vi "autonSample.vi"(0 "Auton Array":dbl[][](array[numeric]), 5 "LeftEncoder":dbl, 7 "RightEncoder":dbl, 11 "MeasuredHeading":dbl) -> (4 "Left Drive":dbl, 6 "Right Drive":dbl, 8 "Ramp ACT motor":dbl, 10 "Harvester":dbl, 13 "Shooter motor output":dbl, 14 "Turret Rotation":dbl, 15 "Convyeor":dbl)   [LabVIEW 2011]
uses:
  Robot Global Data.vi
panel:
  out "Primitive ID":i16
  out "Tzero":i64
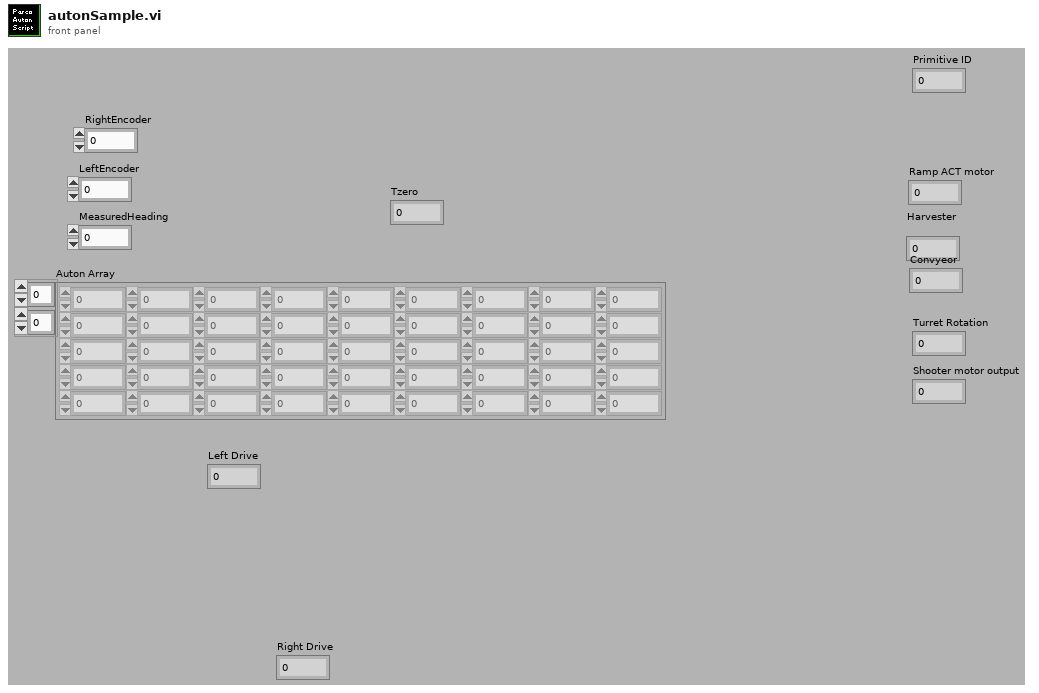
[diagram p1: front panel]
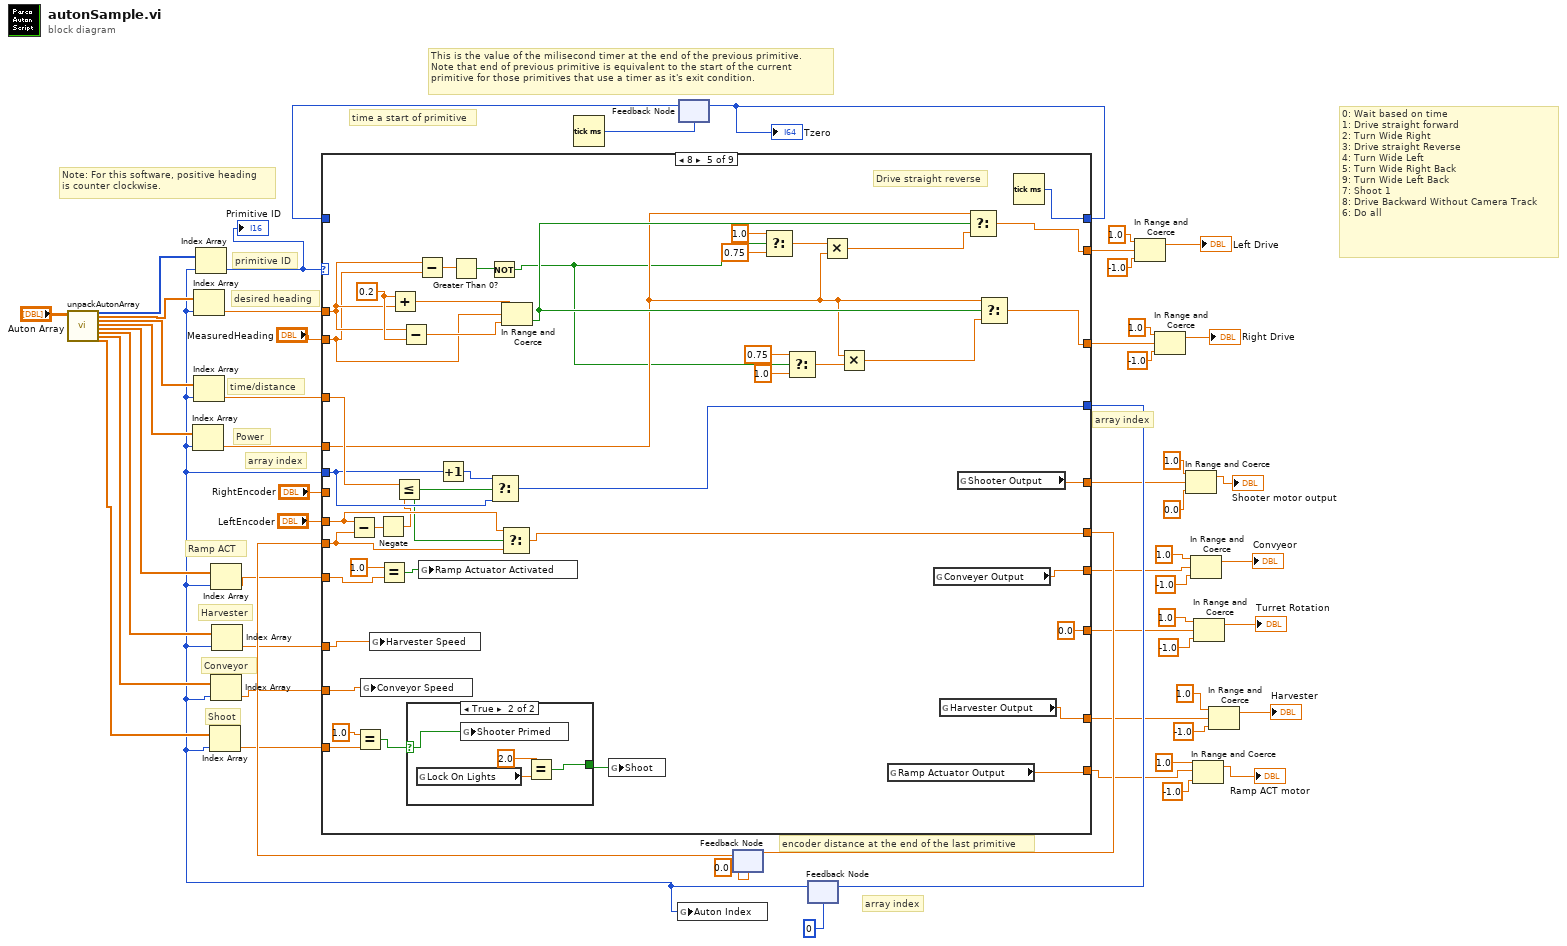
[diagram p0: block diagram]
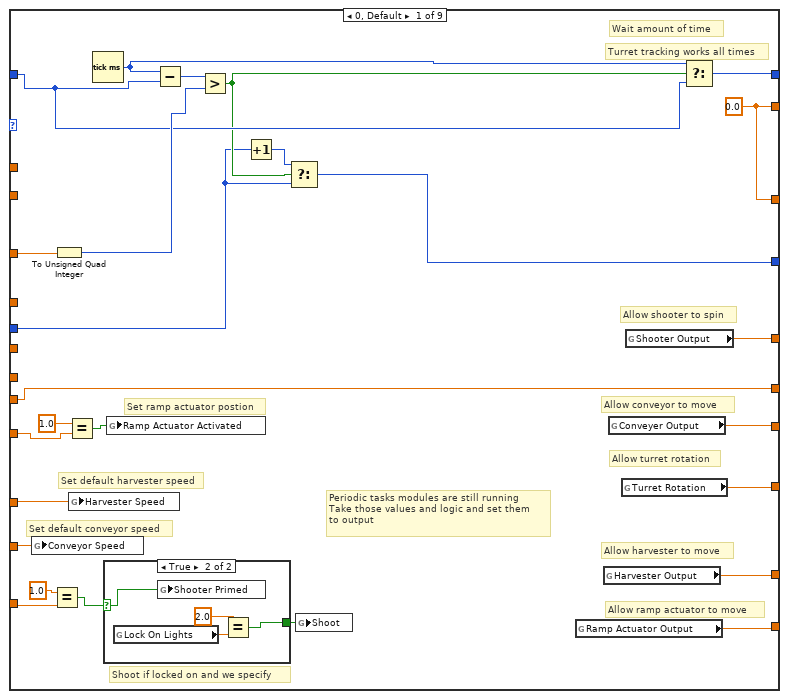
[diagram p2: hidden frame]
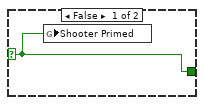
[diagram p3: hidden frame]
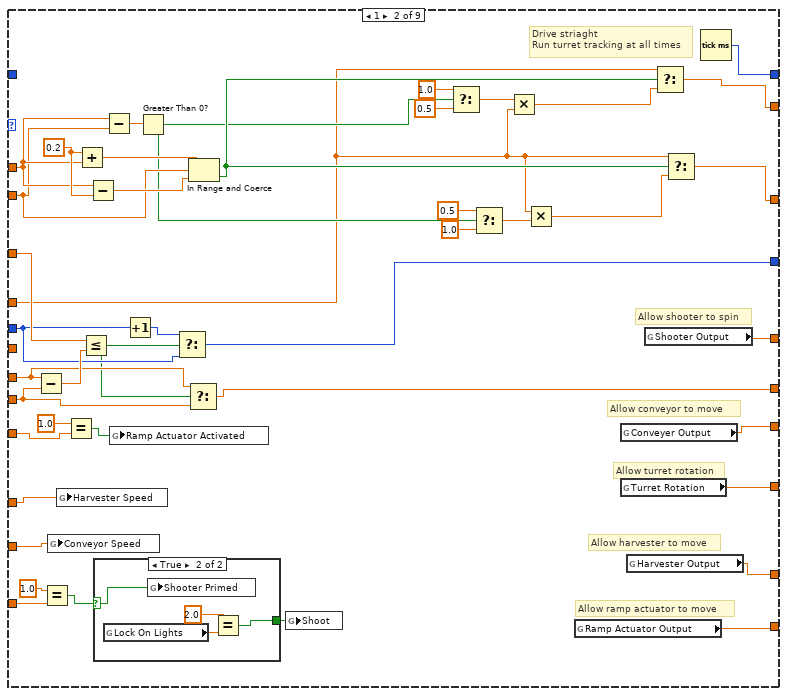
[diagram p4: hidden frame]
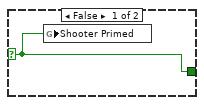
[diagram p5: hidden frame]
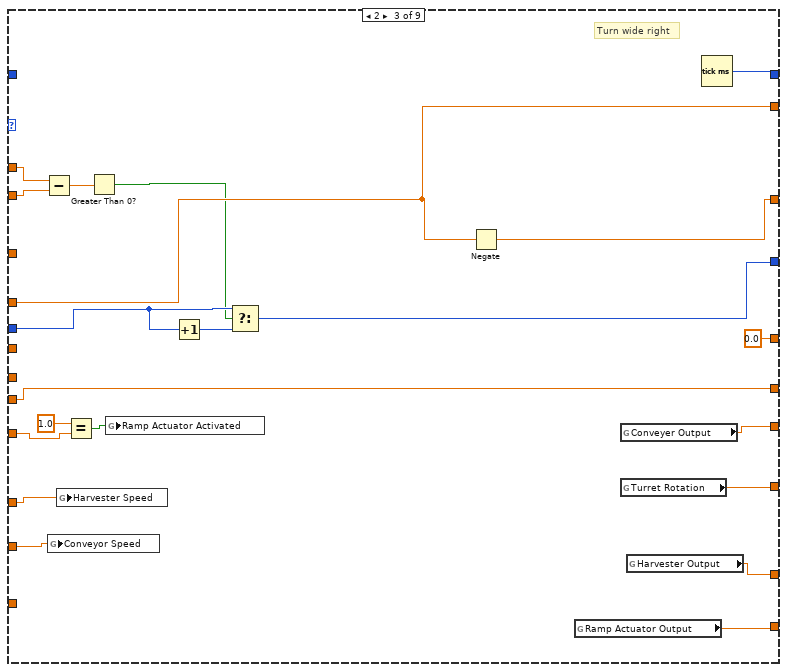
[diagram p6: hidden frame]
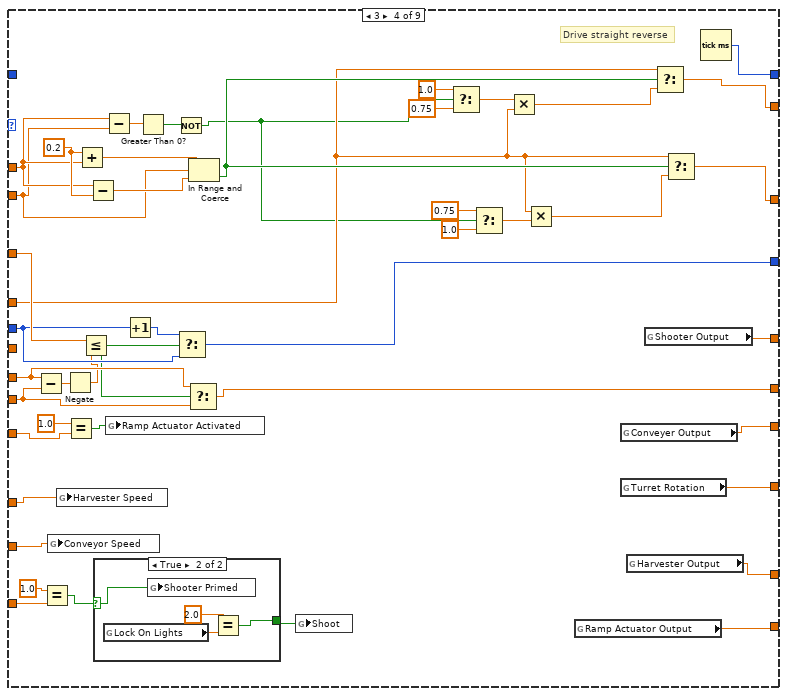
[diagram p7: hidden frame]
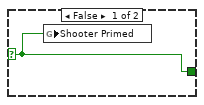
[diagram p8: hidden frame]
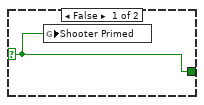
[diagram p9: hidden frame]
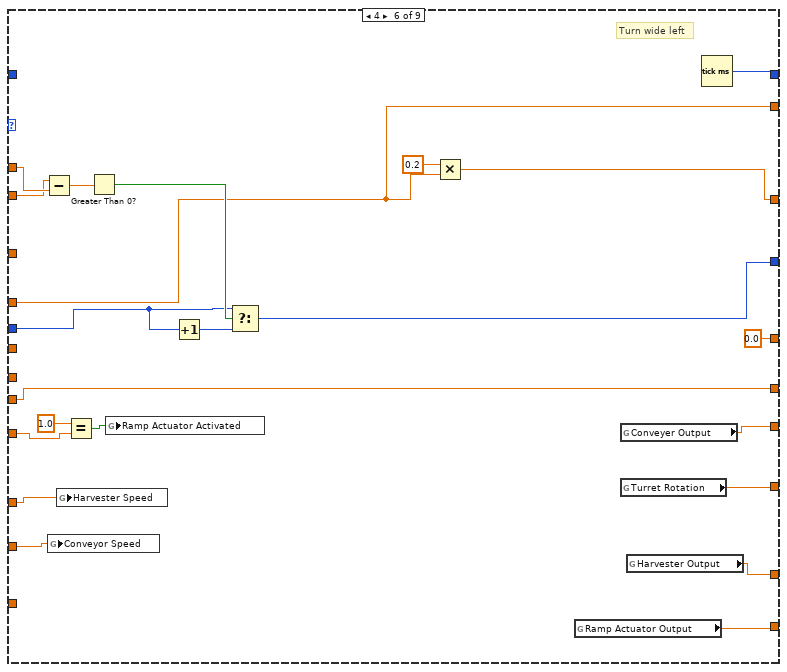
[diagram p10: hidden frame]
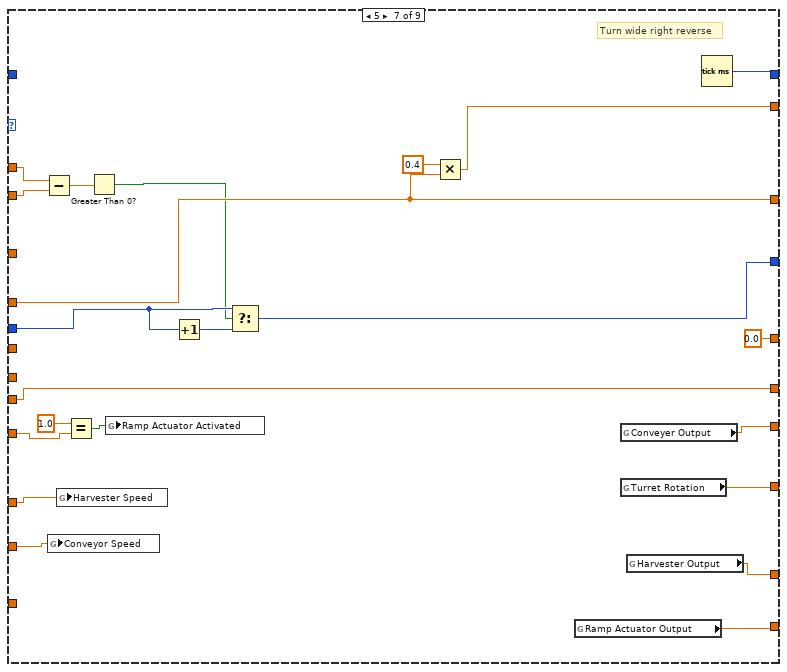
[diagram p11: hidden frame]
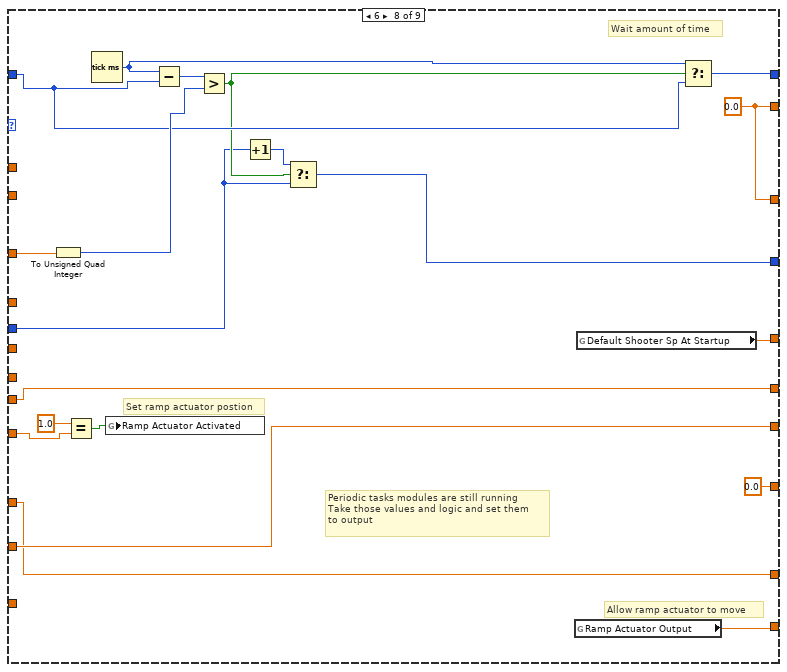
[diagram p12: hidden frame]
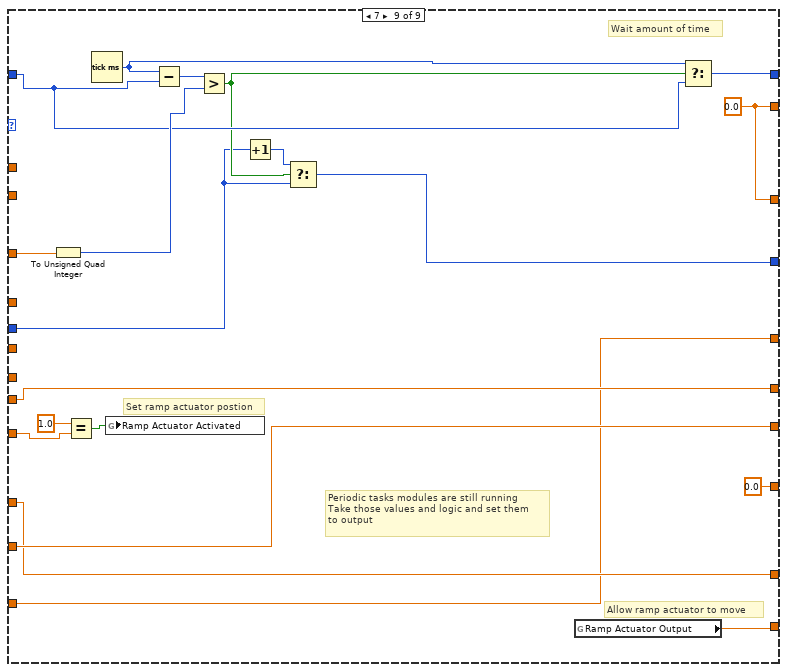
[diagram p13: hidden frame]
diagram:
  # "0: Wait based on time\n1: Drive straight forward\n2: Turn Wide Right\n3: Drive straight Reverse\n4: Turn Wide Left\n5: Turn Wide Right Back\n9: Turn Wide Left Back\n7: Shoot 1\n8: Drive Backward Without Camera Track\n6: Do all"
  # "Shoot"
  # "Conveyor"
  # "Harvester"
  # "Ramp ACT"
  # "encoder distance at the end of the last primitive"
  # "Note: For this software, positive heading\nis counter clockwise."
  # "time a start of primitive"
  # "array index"
  # "array index"
  # "This is the value of the milisecond timer at the end of the previous primitive.\nNote that end of previous primitive is equivalent to the start of the current\nprimitive for those primitives that use a timer as it's exit condition."
  # "Power"
  # "array index"
  # "desired heading"
  # "primitive ID"
  # "time/distance"
  n1 = call "unpackAutonArray.vi"("all rows"="Auton Array") -> ("Primitive"=w56:i16[], "Desired Heading"=w16:dbl[], "Time/Distance"=w15:dbl[], "Power"=w14:dbl[], "Ramp Actuator"=w13:dbl[], "Harvester"=w12:dbl[], "Conveyor"=w11:dbl[], "Shoot"=w10:dbl[])  [unwired: 1 in, 18 out]
  n2 = Tick Count (ms)() -> (millisecond timer value=w51:u32)
  n3 = feedback #1(w51) -> (w55:u32)
  n4 = feedback #2(0.0 ("EncoderDistance")) -> (w39:dbl)
  n5 = feedback #3(0) -> (w8:i32)
  n6 = Index Array(array=w14, index=w8) -> (element=w53:dbl)
  n7 = Index Array(array=w16, index=w8) -> (element=w40:dbl)
  n8 = Index Array(array=w15, index=w8) -> (element=w54:dbl)
  n9 = Index Array(array=w56, index=w8) -> (element=w22:i16)
  "Primitive ID" <- w22
  n10 = Index Array(array=w10, index=w8) -> (element=w9:dbl)
  n11 = Index Array(array=w13, index=w8) -> (element=w21:dbl)
  n12 = Index Array(array=w11, index=w8) -> (element=w6:dbl)
  n13 = Index Array(array=w12, index=w8) -> (element=w7:dbl)
  n14 = case shown="8" w22 {
    tunnel: [w75 w114 w140 w186 w237 w263 w281 w313 w333] -> w35
    tunnel: w8 -> [w76 w116 w142 w188 w239 w265 w283 w314 w334]
    tunnel: [w83 w92 w146 w165 w216 w269 w290 w321 w341] -> w41
    tunnel: w55 -> [w80 _ _ _ _ _ _ w318 w338]
    tunnel: w54 -> [w69 w117 _ w189 w240 _ _ w308 w328]
    tunnel: w40 -> [_ w105 w145 w177 w228 w260 w289 _ _]
    tunnel: [w74 w91 w139 w164 w215 w262 w285 w312 w332] -> w49
    tunnel: [w74 w90 w138 w163 w214 w261 w287 w312 w332] -> w42
    tunnel: w53 -> [_ w94 w139 w167 w218 w262 w287 _ _]
    tunnel: "LeftEncoder" -> [_ w111 _ w183 w234 _ _ _ _]
    tunnel: "MeasuredHeading" -> [_ w104 w144 w176 w227 w259 w288 _ _]
    tunnel: [w68 w113 w148 w185 w236 w271 w292 w307 w327] -> w36
    tunnel: w39 -> [w68 w112 w148 w184 w235 w271 w292 w307 w327]
    tunnel: [w58 w119 0.0 ("Shooter Output") w190 w241 0.0 ("Shooter Output") 0.0 ("Shooter Output") w302 w322] -> w31
    tunnel: [w70 w129 w154 w199 0.0 ("Turret Rotation") w276 w298 0.0 ("Turret Rotation") 0.0 ("Turret Rotation")] -> w27
    tunnel: [w66 w123 w150 w194 w245 w273 w294 w304 w324] -> w23
    tunnel: w21 -> [w63 w126 w153 w162 w213 w258 w297 w306 w326]
    tunnel: [w71 w130 w155 w200 w250 w277 w299 w309 w329] -> w20
    tunnel: w9 -> [w59 w127 _ w197 w248 _ _ _ w322]
    tunnel: w7 -> [w64 w125 w152 w196 w247 w275 w296 w304 w324]
    tunnel: w6 -> [w65 w124 w151 w195 w246 w274 w295 w305 w325]
    tunnel: [w67 w122 w149 w193 w244 w272 w293 w305 w325] -> w2
    tunnel: "RightEncoder" -> [_ _ _ _ _ _ _ _ _]
    frame 0, Default {
      w74 = 0.0 ("Numeric")
      # "Periodic tasks modules are still running\nTake those values and logic and set them \nto output"
      # "Set ramp actuator postion"
      # "Set default harvester speed"
      # "Set default conveyor speed"
      # "Shoot if locked on and we specify"
      # "Allow ramp actuator to move"
      # "Allow harvester to move"
      # "Turret tracking works all times"
      # "Allow turret rotation"
      # "Allow conveyor to move"
      # "Allow shooter to spin"
      # "Wait amount of time"
      n15 = global write "Robot Global Data.vi" "Conveyor Speed"(w65) -> ()
      n16 = Equal?(x=1.0, y=w59) -> (x = y?=w61:bool)
      n17 = To Unsigned Quad Integer(1:w69) -> (0:w81:u64)
      n18 = Equal?(x=1.0, y=w63) -> (x = y?=w72:bool)
      n19 = global write "Robot Global Data.vi" "Harvester Speed"(w64) -> ()
      n20 = Tick Count (ms)() -> (millisecond timer value=w79:u32)
      n21 = case shown="True" w61 {
        selector: w61 -> [w84 w88]
        tunnel: [w84 w85] -> w60
        frame False {
          n22 = global write "Robot Global Data.vi" "Shooter Primed"(w84) -> ()
        }
        frame True {
          n23 = global read "Robot Global Data.vi" "Lock On Lights"() -> (w86:dbl)
          n24 = global write "Robot Global Data.vi" "Shooter Primed"(w88) -> ()
          n25 = Equal?(x=2.0, y=w86) -> (x = y?=w85:bool)
        }
      }
      n26 = global write "Robot Global Data.vi" "Ramp Actuator Activated"(w72) -> ()
      n27 = Subtract(x=w79, y=w80) -> (x-y=w82:u32)
      n28 = Greater?(x=w82, y=w81) -> (0:w78:bool)
      n29 = Increment(x=w76) -> (x+1=w77:i32)
      n30 = Select(t=w77, s=w78, f=w76) -> (s? t:f=w75:i32)
      n31 = global write "Robot Global Data.vi" "Shoot"(w60) -> ()
      n32 = global read "Robot Global Data.vi" "Ramp Actuator Output"() -> (w71:dbl)
      n33 = global read "Robot Global Data.vi" "Harvester Output"() -> (w66:dbl)
      n34 = global read "Robot Global Data.vi" "Conveyer Output"() -> (w67:dbl)
      n35 = global read "Robot Global Data.vi" "Turret Rotation"() -> (w70:dbl)
      n36 = global read "Robot Global Data.vi" "Shooter Output"() -> (w58:dbl)
      n37 = Select(t=w79, s=w78, f=w80) -> (s? t:f=w83:u32)
    }
    frame 1 {
      w109 = 0.2 ("x")
      # "Allow ramp actuator to move"
      # "Allow harvester to move"
      # "Allow turret rotation"
      # "Allow conveyor to move"
      # "Allow shooter to spin"
      # "Drive striaght\nRun turret tracking at all times"
      n38 = Subtract(x=w111, y=w112) -> (x-y=w118:dbl)
      n39 = Equal?(x=1.0, y=w127) -> (x = y?=w121:bool)
      n40 = global write "Robot Global Data.vi" "Conveyor Speed"(w124) -> ()
      n41 = global write "Robot Global Data.vi" "Harvester Speed"(w125) -> ()
      n42 = Equal?(x=1.0, y=w126) -> (x = y?=w89:bool)
      n43 = Add(x=w109, y=w105) -> (x+y=w107:dbl)
      n44 = Less Or Equal?(x=w117, y=w118) -> (x <= y?=w110:bool)
      n45 = Subtract(x=w105, y=w109) -> (x-y=w108:dbl)
      n46 = case shown="True" w121 {
        selector: w121 -> [w132 w136]
        tunnel: [w132 w133] -> w120
        frame False {
          n47 = global write "Robot Global Data.vi" "Shooter Primed"(w132) -> ()
        }
        frame True {
          n48 = global read "Robot Global Data.vi" "Lock On Lights"() -> (w134:dbl)
          n49 = global write "Robot Global Data.vi" "Shooter Primed"(w136) -> ()
          n50 = Equal?(x=2.0, y=w134) -> (x = y?=w133:bool)
        }
      }
      n51 = Subtract(x=w105, y=w104) -> (x-y=w103:dbl)
      n52 = global write "Robot Global Data.vi" "Ramp Actuator Activated"(w89) -> ()
      n53 = Increment(x=w116) -> (x+1=w115:i32)
      n54 = Greater Than 0?(x=w103) -> (x > 0?=w102:bool)
      n55 = Select(t=w115, s=w110, f=w116) -> (s? t:f=w114:i32)
      n56 = Select(t=w111, s=w110, f=w112) -> (s? t:f=w113:dbl)
      n57 = In Range and Coerce(upper limit=w107, x=w104, lower limit=w108) -> (In Range?=w106:bool)  [unwired: 1 out]
      n58 = global write "Robot Global Data.vi" "Shoot"(w120) -> ()
      n59 = Select(t=1.0, s=w102, f=0.5) -> (s? t:f=w95:dbl)
      n60 = Select(t=0.5, s=w102, f=1.0) -> (s? t:f=w97:dbl)
      n61 = Multiply(x=w95, y=w94) -> (x*y=w93:dbl)
      n62 = Multiply(x=w94, y=w97) -> (x*y=w96:dbl)
      n63 = global read "Robot Global Data.vi" "Ramp Actuator Output"() -> (w130:dbl)
      n64 = global read "Robot Global Data.vi" "Conveyer Output"() -> (w122:dbl)
      n65 = global read "Robot Global Data.vi" "Turret Rotation"() -> (w129:dbl)
      n66 = global read "Robot Global Data.vi" "Harvester Output"() -> (w123:dbl)
      n67 = global read "Robot Global Data.vi" "Shooter Output"() -> (w119:dbl)
      n68 = Select(t=w94, s=w106, f=w93) -> (s? t:f=w91:dbl)
      n69 = Select(t=w94, s=w106, f=w96) -> (s? t:f=w90:dbl)
      n70 = Tick Count (ms)() -> (millisecond timer value=w92:u32)
    }
    frame 2 {
      # "Turn wide right"
      n71 = Subtract(x=w145, y=w144) -> (x-y=w143:dbl)
      n72 = global write "Robot Global Data.vi" "Conveyor Speed"(w151) -> ()
      n73 = global write "Robot Global Data.vi" "Harvester Speed"(w152) -> ()
      n74 = Equal?(x=1.0, y=w153) -> (x = y?=w156:bool)
      n75 = Greater Than 0?(x=w143) -> (x > 0?=w137:bool)
      n76 = global write "Robot Global Data.vi" "Ramp Actuator Activated"(w156) -> ()
      n77 = Increment(x=w142) -> (x+1=w141:i32)
      n78 = Select(t=w142, s=w137, f=w141) -> (s? t:f=w140:i32)
      n79 = Negate(x=w139) -> (-x=w138:dbl)
      n80 = global read "Robot Global Data.vi" "Ramp Actuator Output"() -> (w155:dbl)
      n81 = global read "Robot Global Data.vi" "Conveyer Output"() -> (w149:dbl)
      n82 = global read "Robot Global Data.vi" "Turret Rotation"() -> (w154:dbl)
      n83 = global read "Robot Global Data.vi" "Harvester Output"() -> (w150:dbl)
      n84 = Tick Count (ms)() -> (millisecond timer value=w146:u32)
    }
    frame 3 {
      w181 = 0.2 ("x")
      # "Drive straight reverse"
      n85 = Subtract(x=w183, y=w184) -> (x-y=w161:dbl)
      n86 = Equal?(x=1.0, y=w197) -> (x = y?=w192:bool)
      n87 = global write "Robot Global Data.vi" "Conveyor Speed"(w195) -> ()
      n88 = global write "Robot Global Data.vi" "Harvester Speed"(w196) -> ()
      n89 = Negate(x=w161) -> (-x=w160:dbl)
      n90 = Equal?(x=1.0, y=w162) -> (x = y?=w201:bool)
      n91 = Add(x=w181, y=w177) -> (x+y=w179:dbl)
      n92 = Less Or Equal?(x=w189, y=w160) -> (x <= y?=w182:bool)
      n93 = Subtract(x=w177, y=w181) -> (x-y=w180:dbl)
      n94 = case shown="True" w192 {
        selector: w192 -> [w203 w207]
        tunnel: [w203 w204] -> w191
        frame False {
          n95 = global write "Robot Global Data.vi" "Shooter Primed"(w203) -> ()
        }
        frame True {
          n96 = global read "Robot Global Data.vi" "Lock On Lights"() -> (w205:dbl)
          n97 = global write "Robot Global Data.vi" "Shooter Primed"(w207) -> ()
          n98 = Equal?(x=2.0, y=w205) -> (x = y?=w204:bool)
        }
      }
      n99 = Subtract(x=w177, y=w176) -> (x-y=w175:dbl)
      n100 = global write "Robot Global Data.vi" "Ramp Actuator Activated"(w201) -> ()
      n101 = Increment(x=w188) -> (x+1=w187:i32)
      n102 = Greater Than 0?(x=w175) -> (x > 0?=w159:bool)
      n103 = Not(x=w159) -> (.not. x?=w158:bool)
      n104 = Select(t=w187, s=w182, f=w188) -> (s? t:f=w186:i32)
      n105 = Select(t=w183, s=w182, f=w184) -> (s? t:f=w185:dbl)
      n106 = In Range and Coerce(upper limit=w179, x=w176, lower limit=w180) -> (In Range?=w178:bool)  [unwired: 1 out]
      n107 = global write "Robot Global Data.vi" "Shoot"(w191) -> ()
      n108 = Select(t=1.0, s=w158, f=0.75) -> (s? t:f=w168:dbl)
      n109 = Select(t=0.75, s=w158, f=1.0) -> (s? t:f=w170:dbl)
      n110 = Multiply(x=w168, y=w167) -> (x*y=w166:dbl)
      n111 = Multiply(x=w167, y=w170) -> (x*y=w169:dbl)
      n112 = global read "Robot Global Data.vi" "Ramp Actuator Output"() -> (w200:dbl)
      n113 = global read "Robot Global Data.vi" "Conveyer Output"() -> (w193:dbl)
      n114 = global read "Robot Global Data.vi" "Turret Rotation"() -> (w199:dbl)
      n115 = global read "Robot Global Data.vi" "Harvester Output"() -> (w194:dbl)
      n116 = global read "Robot Global Data.vi" "Shooter Output"() -> (w190:dbl)
      n117 = Select(t=w167, s=w178, f=w166) -> (s? t:f=w164:dbl)
      n118 = Select(t=w167, s=w178, f=w169) -> (s? t:f=w163:dbl)
      n119 = Tick Count (ms)() -> (millisecond timer value=w165:u32)
    }
    frame 8 {
      w232 = 0.2 ("x")
      # "Drive straight reverse"
      n120 = Subtract(x=w234, y=w235) -> (x-y=w212:dbl)
      n121 = Equal?(x=1.0, y=w248) -> (x = y?=w243:bool)
      n122 = global write "Robot Global Data.vi" "Conveyor Speed"(w246) -> ()
      n123 = global write "Robot Global Data.vi" "Harvester Speed"(w247) -> ()
      n124 = Negate(x=w212) -> (-x=w211:dbl)
      n125 = Equal?(x=1.0, y=w213) -> (x = y?=w251:bool)
      n126 = Add(x=w232, y=w228) -> (x+y=w230:dbl)
      n127 = Less Or Equal?(x=w240, y=w211) -> (x <= y?=w233:bool)
      n128 = Subtract(x=w228, y=w232) -> (x-y=w231:dbl)
      n129 = case shown="True" w243 {
        selector: w243 -> [w253 w257]
        tunnel: [w253 w254] -> w242
        frame False {
          n130 = global write "Robot Global Data.vi" "Shooter Primed"(w253) -> ()
        }
        frame True {
          n131 = global read "Robot Global Data.vi" "Lock On Lights"() -> (w255:dbl)
          n132 = global write "Robot Global Data.vi" "Shooter Primed"(w257) -> ()
          n133 = Equal?(x=2.0, y=w255) -> (x = y?=w254:bool)
        }
      }
      n134 = Subtract(x=w228, y=w227) -> (x-y=w226:dbl)
      n135 = global write "Robot Global Data.vi" "Ramp Actuator Activated"(w251) -> ()
      n136 = Increment(x=w239) -> (x+1=w238:i32)
      n137 = Greater Than 0?(x=w226) -> (x > 0?=w210:bool)
      n138 = Not(x=w210) -> (.not. x?=w209:bool)
      n139 = Select(t=w238, s=w233, f=w239) -> (s? t:f=w237:i32)
      n140 = Select(t=w234, s=w233, f=w235) -> (s? t:f=w236:dbl)
      n141 = In Range and Coerce(upper limit=w230, x=w227, lower limit=w231) -> (In Range?=w229:bool)  [unwired: 1 out]
      n142 = global write "Robot Global Data.vi" "Shoot"(w242) -> ()
      n143 = Select(t=1.0, s=w209, f=0.75) -> (s? t:f=w219:dbl)
      n144 = Select(t=0.75, s=w209, f=1.0) -> (s? t:f=w221:dbl)
      n145 = Multiply(x=w219, y=w218) -> (x*y=w217:dbl)
      n146 = Multiply(x=w218, y=w221) -> (x*y=w220:dbl)
      n147 = global read "Robot Global Data.vi" "Ramp Actuator Output"() -> (w250:dbl)
      n148 = global read "Robot Global Data.vi" "Conveyer Output"() -> (w244:dbl)
      n149 = global read "Robot Global Data.vi" "Harvester Output"() -> (w245:dbl)
      n150 = global read "Robot Global Data.vi" "Shooter Output"() -> (w241:dbl)
      n151 = Select(t=w218, s=w229, f=w217) -> (s? t:f=w215:dbl)
      n152 = Select(t=w218, s=w229, f=w220) -> (s? t:f=w214:dbl)
      n153 = Tick Count (ms)() -> (millisecond timer value=w216:u32)
    }
    frame 4 {
      # "Turn wide left"
      n154 = Subtract(x=w259, y=w260) -> (x-y=w267:dbl)
      n155 = global write "Robot Global Data.vi" "Conveyor Speed"(w274) -> ()
      n156 = global write "Robot Global Data.vi" "Harvester Speed"(w275) -> ()
      n157 = Equal?(x=1.0, y=w258) -> (x = y?=w278:bool)
      n158 = Greater Than 0?(x=w267) -> (x > 0?=w266:bool)
      n159 = global write "Robot Global Data.vi" "Ramp Actuator Activated"(w278) -> ()
      n160 = Increment(x=w265) -> (x+1=w264:i32)
      n161 = Select(t=w265, s=w266, f=w264) -> (s? t:f=w263:i32)
      n162 = Multiply(x=0.2, y=w262) -> (x*y=w261:dbl)
      n163 = global read "Robot Global Data.vi" "Ramp Actuator Output"() -> (w277:dbl)
      n164 = global read "Robot Global Data.vi" "Conveyer Output"() -> (w272:dbl)
      n165 = global read "Robot Global Data.vi" "Turret Rotation"() -> (w276:dbl)
      n166 = global read "Robot Global Data.vi" "Harvester Output"() -> (w273:dbl)
      n167 = Tick Count (ms)() -> (millisecond timer value=w269:u32)
    }
    frame 5 {
      # "Turn wide right reverse"
      n168 = Subtract(x=w289, y=w288) -> (x-y=w284:dbl)
      n169 = global write "Robot Global Data.vi" "Conveyor Speed"(w295) -> ()
      n170 = global write "Robot Global Data.vi" "Harvester Speed"(w296) -> ()
      n171 = Equal?(x=1.0, y=w297) -> (x = y?=w300:bool)
      n172 = Greater Than 0?(x=w284) -> (x > 0?=w280:bool)
      n173 = global write "Robot Global Data.vi" "Ramp Actuator Activated"(w300) -> ()
      n174 = Increment(x=w283) -> (x+1=w282:i32)
      n175 = Select(t=w283, s=w280, f=w282) -> (s? t:f=w281:i32)
      n176 = Multiply(x=0.4, y=w287) -> (x*y=w285:dbl)
      n177 = global read "Robot Global Data.vi" "Ramp Actuator Output"() -> (w299:dbl)
      n178 = global read "Robot Global Data.vi" "Conveyer Output"() -> (w293:dbl)
      n179 = global read "Robot Global Data.vi" "Turret Rotation"() -> (w298:dbl)
      n180 = global read "Robot Global Data.vi" "Harvester Output"() -> (w294:dbl)
      n181 = Tick Count (ms)() -> (millisecond timer value=w290:u32)
    }
    frame 6 {
      w312 = 0.0 ("Numeric")
      # "Periodic tasks modules are still running\nTake those values and logic and set them \nto output"
      # "Set ramp actuator postion"
      # "Allow ramp actuator to move"
      # "Wait amount of time"
      n182 = To Unsigned Quad Integer(1:w308) -> (0:w319:u64)
      n183 = Equal?(x=1.0, y=w306) -> (x = y?=w310:bool)
      n184 = Tick Count (ms)() -> (millisecond timer value=w317:u32)
      n185 = global write "Robot Global Data.vi" "Ramp Actuator Activated"(w310) -> ()
      n186 = Subtract(x=w317, y=w318) -> (x-y=w320:u32)
      n187 = Greater?(x=w320, y=w319) -> (0:w316:bool)
      n188 = Increment(x=w314) -> (x+1=w315:i32)
      n189 = Select(t=w315, s=w316, f=w314) -> (s? t:f=w313:i32)
      n190 = global read "Robot Global Data.vi" "Ramp Actuator Output"() -> (w309:dbl)
      n191 = global read "Robot Global Data.vi" "Default Shooter Sp At Startup"() -> (w302:dbl)
      n192 = Select(t=w317, s=w316, f=w318) -> (s? t:f=w321:u32)
    }
    frame 7 {
      w332 = 0.0 ("Numeric")
      # "Periodic tasks modules are still running\nTake those values and logic and set them \nto output"
      # "Set ramp actuator postion"
      # "Allow ramp actuator to move"
      # "Wait amount of time"
      n193 = To Unsigned Quad Integer(1:w328) -> (0:w339:u64)
      n194 = Equal?(x=1.0, y=w326) -> (x = y?=w330:bool)
      n195 = Tick Count (ms)() -> (millisecond timer value=w337:u32)
      n196 = global write "Robot Global Data.vi" "Ramp Actuator Activated"(w330) -> ()
      n197 = Subtract(x=w337, y=w338) -> (x-y=w340:u32)
      n198 = Greater?(x=w340, y=w339) -> (0:w336:bool)
      n199 = Increment(x=w334) -> (x+1=w335:i32)
      n200 = Select(t=w335, s=w336, f=w334) -> (s? t:f=w333:i32)
      n201 = global read "Robot Global Data.vi" "Ramp Actuator Output"() -> (w329:dbl)
      n202 = Select(t=w337, s=w336, f=w338) -> (s? t:f=w341:u32)
    }
  }
  "Tzero" <- w41
  n203 = global write "Robot Global Data.vi" "Auton Index"(w8) -> ()
  n204 = feedback-in #1(w41) -> ()
  n205 = feedback-in #2(w36) -> ()
  n206 = feedback-in #3(w35) -> ()
  n207 = In Range and Coerce(upper limit=1.0, x=w49, lower limit=-1.0) -> (coerced(x)=→"Left Drive":dbl)  [unwired: 1 out]
  n208 = In Range and Coerce(upper limit=1.0, x=w42, lower limit=-1.0) -> (coerced(x)=→"Right Drive":dbl)  [unwired: 1 out]
  n209 = In Range and Coerce(upper limit=1.0, x=w31, lower limit=0.0) -> (coerced(x)=→"Shooter motor output":dbl)  [unwired: 1 out]
  n210 = In Range and Coerce(upper limit=1.0, x=w2, lower limit=-1.0) -> (coerced(x)=→"Convyeor":dbl)  [unwired: 1 out]
  n211 = In Range and Coerce(upper limit=1.0, x=w20, lower limit=-1.0) -> (coerced(x)=→"Ramp ACT motor":dbl)  [unwired: 1 out]
  n212 = In Range and Coerce(upper limit=1.0, x=w27, lower limit=-1.0) -> (coerced(x)=→"Turret Rotation":dbl)  [unwired: 1 out]
  n213 = In Range and Coerce(upper limit=1.0, x=w23, lower limit=-1.0) -> (coerced(x)=→"Harvester":dbl)  [unwired: 1 out]
